vi "BuildSpecifications.vi"(6 "ItemBuilt":T2, 8 "error in (no error)":errorcluster, 11 "SolutionBuilder in":refnum<class "SolutionBuilder.lvclass">) -> (0 "error out":errorcluster, 1 "Generated files":T1[](array[typedef]), 3 "SolutionBuilder out":refnum<class "SolutionBuilder.lvclass">)   [LabVIEW 2020, in "SolutionBuilder.lvlib" / "SolutionBuilder.lvclass"]
uses:
  SolutionBuilder.lvclass
  Events/EventItemBuilt.ctl
  SolutionBuilder.lvclass/SolutionBuilder.ctl
  BuildManager/BuildManager.lvclass
  SolutionBuilder.lvlib
  BuildManager/GeneratedFile.ctl
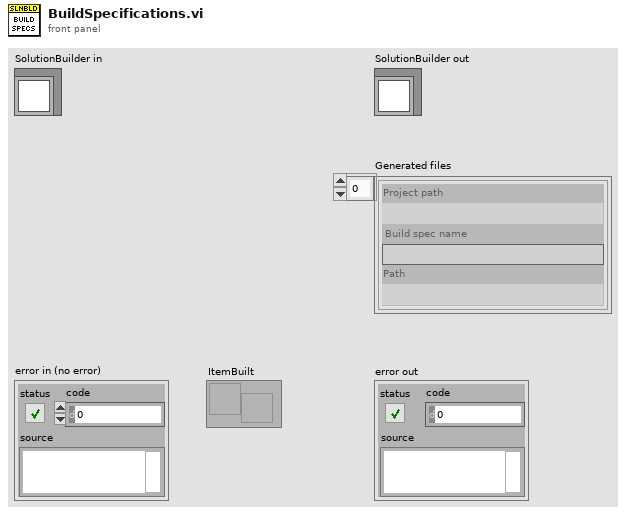
[diagram p1: front panel]
types:
  T1 = typedef "SolutionBuilder.lvlib/BuildManager.lvclass/GeneratedFile.ctl" = cluster{"Project path":path, "Build spec name":string, "Path":path}
  T2 = typedef "SolutionBuilder.lvlib/EventItemBuilt.ctl" = refnum<user-event>
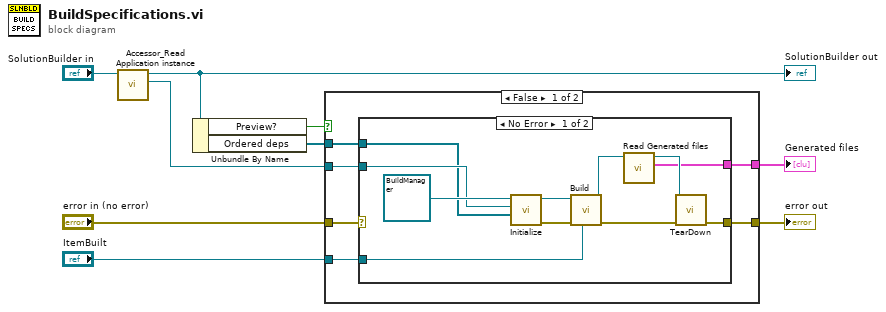
[diagram p0: block diagram]
diagram:
  n1 = call "Accessor_Read Application instance.vi"("SolutionBuilder in"="SolutionBuilder in") -> ("App instance"=w2:refnum<vi>, "SolutionBuilder out"=w3:refnum<class "SolutionBuilder.lvclass">)  [unwired: 8 in, 1 out]
  "SolutionBuilder out" <- w3
  n2 = Unbundle By Name(w3) -> ("Preview?"=w7:bool, "Ordered deps"=w9:refnum<class "ProjectItem.lvclass">[])
  n3 = case shown="False" w7 {
    tunnel: w2 -> [w15 _]
    tunnel: w9 -> [w14 _]
    tunnel: "ItemBuilt" -> [w13 _]
    tunnel: "error in (no error)" -> [w12 w28]
    tunnel: [w11 w28] -> w5
    tunnel: [w10 _] -> w1
    frame False {
      n4 = case shown="No Error" w12 {
        selector: w12 -> [_ w27]
        tunnel: w15 -> [w25 _]
        tunnel: w14 -> [w24 _]
        tunnel: w13 -> [w22 _]
        tunnel: [w19 w27] -> w11
        tunnel: [w16 _] -> w10
        frame No Error {
          n5 = call "Initialize.vi"("Ordered deps"=w24, "Application in"=w25, "BuildManager in"=refnum<class "BuildManager.lvclass"> refnum ("SolutionBuilder.lvlib:BuildManager.lvclass")) -> ("error out"=w20:errorcluster, "BuildManager out"=w23:refnum<class "BuildManager.lvclass">)  [unwired: 7 in]
          n6 = call "Build.vi"("ItemBuilt"=w22, "error in (no error)"=w20, "BuildManager in"=w23) -> ("error out"=w21:errorcluster, "BuildManager out"=w18:refnum<class "BuildManager.lvclass">)  [unwired: 7 in]
          n7 = call-dynamic "Read Generated files.vi"("BuildManager in"=w18) -> ("Generated files"=w16:T1[], "BuildManager out"=w17:refnum<class "BuildManager.lvclass">)  [unwired: 9 in]
          n8 = call "TearDown.vi"("error in (no error)"=w21, "BuildManager in"=w17) -> ("error out"=w19:errorcluster)  [unwired: 8 in, 1 out]
        }
        frame Error {
        }
      }
    }
    frame True {
    }
  }
  "error out" <- w5
  "Generated files" <- w1
